vi "IndentLevel.vi"() -> ()   [LabVIEW 2013]
panel:
  in  "IndentLevel":i32
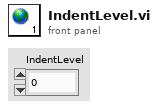
[diagram p1: front panel]
diagram:
